vi "txt_to_roi.vi"(6 "number of frames":i32, 8 "error in (no error)":errorcluster, 10 "path in":path, 11 "TrajectoryMH100122AODRAPS in":refnum<class "TrajectoryMH100122AODRAPS.lvclass">) -> (0 "error out":errorcluster, 2 "output array out":T1(array[cluster]), 3 "TrajectoryMH100122AODRAPS out":refnum<class "TrajectoryMH100122AODRAPS.lvclass">)   [LabVIEW 2010, in "TrajectoryMH100122AODRAPS.lvclass"]
uses:
  TrajectoryMH100122AODRAPS.lvclass
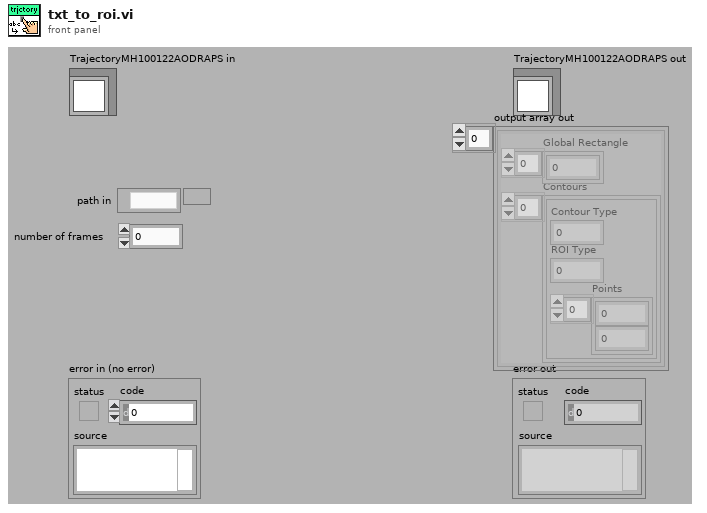
[diagram p1: front panel]
types:
  T1 = cluster{"Global Rectangle":i32[], "Contours":cluster{"Contour Type":u32, "ROI Type":u32, "Points":i32[]}[]}[]
  T2 = cluster{"Global Rectangle":i32[], "Contours":cluster{"Contour Type":u32, "ROI Type":u32, "Points":i32[]}[]}
  T3 = enum16{"open", "replace", "create", "open or create", "replace or create", "replace or create with confirmation"}
  T4 = cluster{"Contour Type":u32, "ROI Type":u32, "Points":i32[]}[]
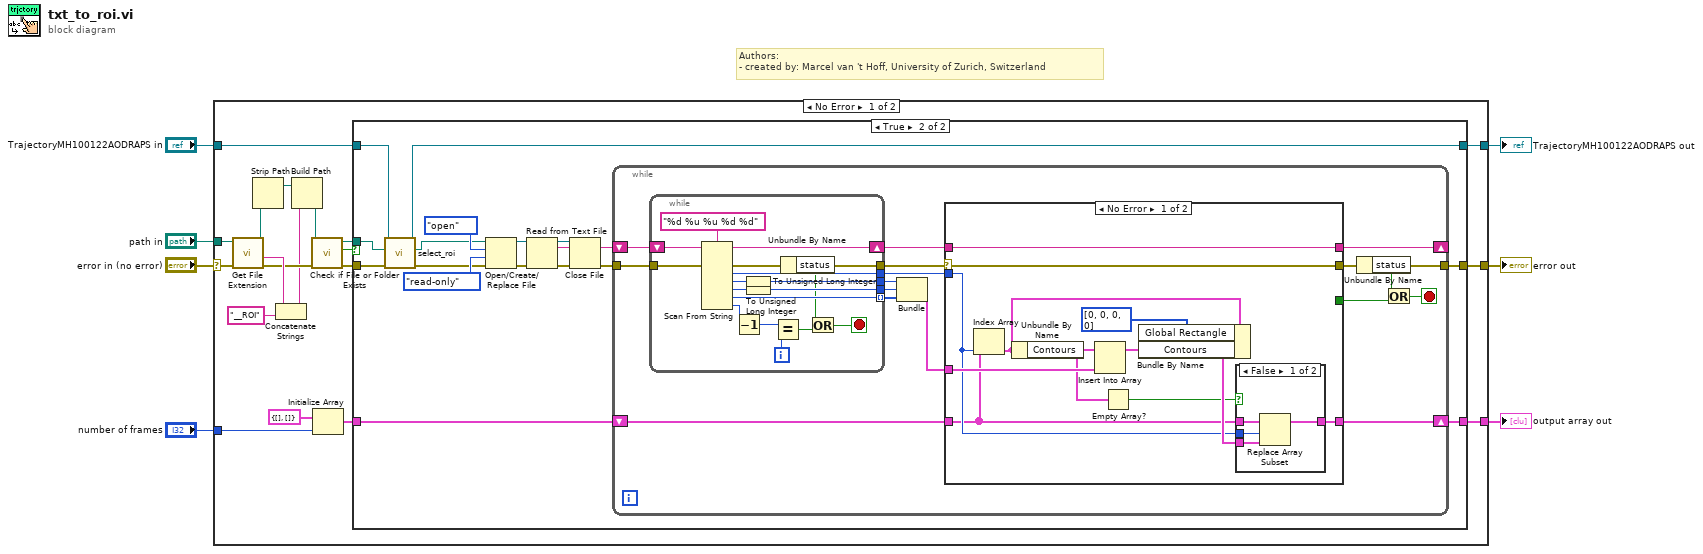
[diagram p0: block diagram]
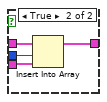
[diagram p3: hidden frame]
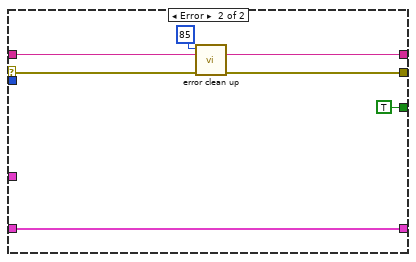
[diagram p4: hidden frame]
diagram:
  # "Authors: \n- created by: Marcel van 't Hoff, University of Zurich, Switzerland"
  n1 = case shown="No Error" "error in (no error)" {
    selector: "error in (no error)" -> [w15 w106]
    tunnel: [w24 w106] -> w6
    tunnel: [w22 w105] -> w4
    tunnel: "TrajectoryMH100122AODRAPS in" -> [w21 w105]
    tunnel: "path in" -> [w16 _]
    tunnel: [w12 _] -> w2
    tunnel: "number of frames" -> [w11 _]
    frame No Error {
      n2 = call <vilib>:"Get File Extension.vi"("error in (no error)"=w15, "file"=w16) -> ("error out"=w14:errorcluster, "filename without extension"=w19:string, "dup file"=w17:path)  [unwired: 6 in, 1 out]
      n3 = Strip Path(path=w17) -> (stripped path=w20:path)  [unwired: 1 out]
      n4 = Concatenate Strings(w19, "__ROI" ("string")) -> (w8:string)
      n5 = Build Path(base path=w20, name or relative path=w8) -> (appended path=w13:path)
      n6 = call <vilib>:"Check if File or Folder Exists.vi"("error in (no error)"=w14, "path"=w13) -> ("error out"=w23:errorcluster, "file or folder exists?"=w26:bool, "dup path"=w25:path)  [unwired: 7 in]
      n7 = Initialize Array(T2 {"Global Rectangle"=[], "Contours"=[]} ("ROI"), w11) -> (w9:T1)
      n8 = case shown="True" w26 {
        tunnel: w25 -> [_ w30]
        tunnel: [w28 w37] -> w24
        tunnel: w23 -> [w28 w32]
        tunnel: [w27 w33] -> w22
        tunnel: w21 -> [w27 w34]
        tunnel: [_ w36] -> w12
        tunnel: w9 -> [_ w35]
        frame False {
        }
        frame True {
          n9 = call-dynamic "select_roi.vi"("error in (no error)"=w32, "path in"=w30, "TrajectoryMH100122AODRAPS in"=w34) -> ("error out"=w31:errorcluster, "selected path out"=w29:path, "TrajectoryMH100122AODRAPS out"=w33:refnum<class "TrajectoryMH100122AODRAPS.lvclass">)  [unwired: 6 in]
          n10 = Open/Create/Replace File(file path (use dialog)=w29, error in=w31, operation (0:open)=T3."open", access (0:read/write)=enum16{"read/write", "read-only", "write-only"}."read-only") -> (refnum out=w42:refnum<file>, error out=w43:errorcluster)  [unwired: 2 in, 1 out]
          n11 = Read from Text File(file (use dialog)=w42, error in=w43) -> (refnum out=w40:refnum<file>, text=w41:string, error out=w39:errorcluster)  [unwired: 2 in, 1 out]
          n12 = Close File(refnum=w40, error in=w39) -> (error out=w38:errorcluster)  [unwired: 1 out]
          n13 = while {
            tunnel: w38 -> [w60]
            tunnel: [w49] -> w37
            shift-right: [w53] -> w36
            shift-left: w35 -> [w54]
            shift-right: [w50] -> _
            shift-left: w41 -> [w61]
            stop <- w48 stop-if-true
            n14 = while {
              tunnel: w60 -> [w77]
              tunnel: [w76] -> w59
              tunnel: [w75] -> w58
              tunnel: [w64] -> w52
              tunnel: [w74] -> w55
              tunnel: [w69] -> w57 mode=indexing
              shift-right: [w73] -> w51
              shift-left: w61 -> [w78]
              i -> [w67]
              stop <- w63 stop-if-true
              n15 = Scan From String(format string="%d %u %u %d %d", input string=w78, error in=w77) -> (remaining string=w73:string, error out=w64:errorcluster, output 1=w74:i32, output 2=w71:i32, output 3=w70:i32, output 4=w69:i32, output 5=w68:i32)  [unwired: 6 in, 1 out]
              n16 = Decrement(x=w68) -> (x-1=w66:i32)
              n17 = To Unsigned Long Integer(number=w71) -> (unsigned 32bit integer=w76:u32)
              n18 = To Unsigned Long Integer(number=w70) -> (unsigned 32bit integer=w75:u32)
              n19 = Equal?(x=w66, y=w67) -> (x = y?=w65:bool)
              n20 = Unbundle By Name(w64) -> ("status"=w62:bool)
              n21 = Or(x=w62, y=w65) -> (x .or. y?=w63:bool)
            }
            n22 = Bundle(w59, w58, w57) -> (w56:cluster{u32, u32, i32[]})  [unwired: 1 in]
            n23 = case shown="No Error" w52 {
              selector: w52 -> [w81 w102]
              tunnel: w56 -> [w90 _]
              tunnel: w55 -> [w87 _]
              tunnel: w54 -> [w86 w104]
              tunnel: [w85 w104] -> w53
              tunnel: [w81 w101] -> w49
              tunnel: [w79 w100] -> w50
              tunnel: w51 -> [w79 w100]
              tunnel: [_ TRUE] -> w46
              frame No Error {
                n24 = Index Array(array=w86, index=w87) -> (element=w84:T2)
                n25 = Unbundle By Name(w84) -> ("Contours"=w83:T4)
                n26 = Insert Into Array(array=w83, new element=w90) -> (w89:T4)  [unwired: 1 in]
                n27 = Empty Array?(array=w83) -> (empty?=w82:bool)
                n28 = Bundle By Name(cluster=w84, "Global Rectangle"=i32[] [0, 0, 0, 0], "Contours"=w89) -> (w88:T2)
                n29 = case shown="False" w82 {
                  tunnel: w88 -> [w94 w95]
                  tunnel: w87 -> [w93 w96]
                  tunnel: w86 -> [w92 w98]
                  tunnel: [w91 w97] -> w85
                  frame False {
                    n30 = Replace Array Subset(array=w92, new element=w94, index=w93) -> (w91:T1)
                  }
                  frame True {
                    n31 = Insert Into Array(array=w98, index=w96, new element=w95) -> (w97:T1)
                  }
                }
              }
              frame Error {
                n32 = call "error clean up.vi"("error in"=w102, "code in"=85) -> ("error out"=w101:errorcluster)  [unwired: 9 in]
              }
            }
            n33 = Unbundle By Name(w49) -> ("status"=w47:bool)
            n34 = Or(x=w47, y=w46) -> (x .or. y?=w48:bool)
          }
        }
      }
    }
    frame Error {
    }
  }
  "error out" <- w6
  "TrajectoryMH100122AODRAPS out" <- w4
  "output array out" <- w2
